vi "Config Type.vi"(11 "Inc Var Command in":refnum<class "Inc Var Command.lvclass">) -> (2 "Command Config Type":refnum<class "Command Config.lvclass">)   [LabVIEW 2020, in "VolatusSeq.lvlib" / "Inc Var Command.lvclass"]
uses:
  Inc Var Command.lvclass
  Inc Var Command.lvclass/Inc Var Command.ctl
  VolatusSeqConfig/Inc Var Command Config/Inc Var Command Config.lvclass
  C:/dev/lv20CE/relink/lv-volatus/VolatusSeqConfig/Command Config/Command Config.lvclass
  C:/dev/lv20CE/relink/lv-volatus/VolatusSeqConfig/Inc Var Command Config/Inc Var Command Config.lvclass
  VolatusSeqConfig/Command Config/Command Config.lvclass
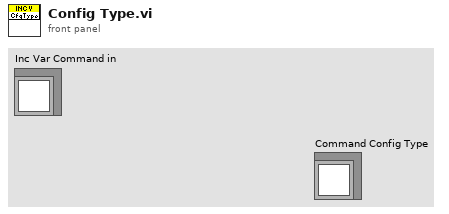
[diagram p1: front panel]
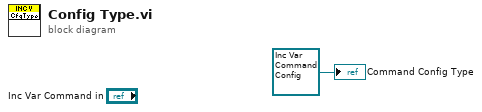
[diagram p0: block diagram]
diagram:
  "Command Config Type" <- refnum<class "Inc Var Command Config.lvclass"> refnum ("VolatusSeqConfig.lvlib:Inc Var Command Config.lvclass")
